vi "Controlled voltage ramp checking current.vi"(6 "Barcodes in":string[](array[string]), 9 "Stop Program":bool, 11 "VISA Refnum in":refnum<visa-resource-name>) -> (0 "error out":errorcluster, 3 "BoardHandle out 2":T1, 10 "Power Supply Trip":bool)   [LabVIEW 2020]
uses:
  <instrlib>/CAEN PSM/CAEN PSM.lvlib
panel:
  out "Actual Voltage Level (V)":dbl format="%#_13g"
  out "Actual Current Limit (nA)":dbl format="%#_13g"
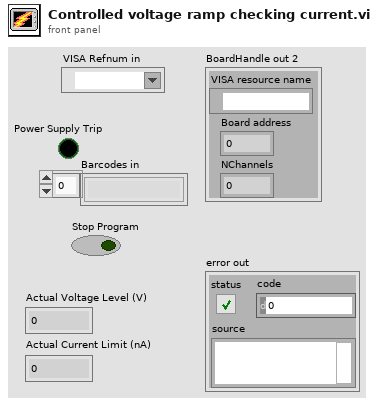
[diagram p1: front panel]
types:
  T1 = cluster{"VISA resource name":refnum<visa-resource-name>, "Board address":u8, "NChannels":u8}
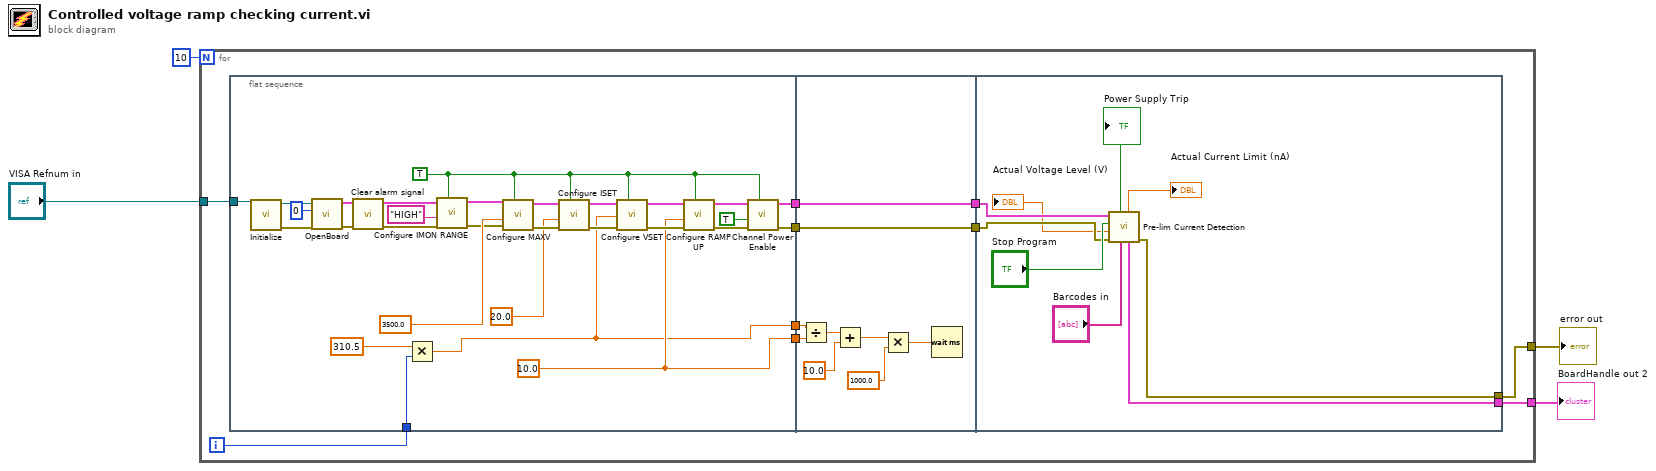
[diagram p0: block diagram]
diagram:
  n1 = for {
    N: 10 -> [_]
    tunnel: "VISA Refnum in" -> [w10]
    tunnel: [w9] -> w3
    tunnel: [w8] -> w2
    i -> [w7]
    n2 = flat-sequence {
      tunnel: [w17] -> w14
      tunnel: [w29] -> w13
      tunnel: [w28] -> w12
      tunnel: [w27] -> w11
      tunnel: w10 -> [w26]
      tunnel: w7 -> [w15]
      tunnel: w14 -> [w47]
      tunnel: w13 -> [w46]
      tunnel: w12 -> [w45]
      tunnel: w11 -> [w44]
      tunnel: [w45] -> w6
      tunnel: [w44] -> w5
      tunnel: [w58] -> w9
      tunnel: [w57] -> w8
      tunnel: w6 -> [w60]
      tunnel: w5 -> [w59]
      frame #0 {
        w19 = TRUE ("All Channels (F)")
        w29 = 10.0 ("Voltage Ramp Up (V/s)")
        n3 = call <instrlib>:"Initialize.vi"("VISA resource name"=w26) -> ("error out"=w38:errorcluster, "VISA resource name out"=w35:refnum<visa-resource-name>)  [unwired: 9 in]
        n4 = call <instrlib>:"OpenBoard.vi"("error in (no error)"=w38, "Board Address"=u8 0, "VISA resource name"=w35) -> ("error out"=w39:errorcluster, "BoardHandle"=w34:T1)  [unwired: 7 in]
        n5 = call <instrlib>:"Clear alarm signal.vi"("error in (no error)"=w39, "BoardHandle"=w34) -> ("error out"=w24:errorcluster, "BoardHandle out"=w23:T1)  [unwired: 8 in]
        n6 = Multiply(x=310.5, y=w15) -> (x*y=w17:dbl)
        n7 = call <instrlib>:"Configure IMON RANGE.vi"("All Channels (F)"=w19, "error in (no error)"=w24, "IMon range (LOW)"="HIGH", "BoardHandle"=w23) -> ("error out"=w20:errorcluster, "BoardHandle out"=w21:T1)  [unwired: 6 in]
        n8 = call <instrlib>:"Configure MAXV.vi"("All Channels (F)"=w19, "error in (no error)"=w20, "Voltage Max (0.0 V)"=3500.0 ("VMax (Volts)"), "BoardHandle"=w21) -> ("error out"=w40:errorcluster, "BoardHandle out"=w33:T1)  [unwired: 6 in]
        n9 = call <instrlib>:"Configure ISET.vi"("All Channels (F)"=w19, "error in (no error)"=w40, "Current Limit (0.00 uA)"=20.0 ("Current Limit (uA)"), "BoardHandle"=w33) -> ("error out"=w41:errorcluster, "BoardHandle out"=w32:T1)  [unwired: 6 in]
        n10 = call <instrlib>:"Configure VSET.vi"("All Channels (F)"=w19, "error in (no error)"=w41, "Voltage Level (0.0 V)"=w17, "BoardHandle"=w32) -> ("error out"=w42:errorcluster, "BoardHandle out"=w31:T1)  [unwired: 6 in]
        n11 = call <instrlib>:"Configure RAMP UP.vi"("All Channels (F)"=w19, "error in (no error)"=w42, "Voltage ramp up (0 V/s)"=w29, "BoardHandle"=w31) -> ("error out"=w43:errorcluster, "BoardHandle out"=w30:T1)  [unwired: 6 in]
        n12 = call <instrlib>:"Channel Power Enable.vi"("All Channels (F)"=w19, "error in (no error)"=w43, "Enable (OFF)"=TRUE ("Boolean"), "BoardHandle"=w30) -> ("error out"=w27:errorcluster, "BoardHandle out"=w28:T1)  [unwired: 6 in]
      }
      frame #1 {
        n13 = Divide(x=w47, y=w46) -> (x/y=w50:dbl)
        n14 = Add(x=w50, y=10.0) -> (x+y=w51:dbl)
        n15 = Multiply(x=w51, y=1000.0) -> (x*y=w52:dbl)
        n16 = Wait (ms)(milliseconds to wait=w52) -> ()  [unwired: 1 out]
      }
      frame #2 {
        n17 = call "Pre-lim Current Detection.vi"("Barcodes in"="Barcodes in", "error in (no error)"=w59, "Stop Program"="Stop Program", "BoardHandle in"=w60) -> ("error out"=w58:errorcluster, "BoardHandle out 3"=w57:T1, "Actual Current Limit (nA)"=→"Actual Current Limit (nA)":dbl, "Power Supply Trip"=→"Power Supply Trip":bool, "Actual Voltage Level (V)"=→"Actual Voltage Level (V)":dbl)  [unwired: 3 out]
      }
    }
  }
  "BoardHandle out 2" <- w2
  "error out" <- w3
